vi "Update_Repeat_Param_Value_SubVI.vi"(10 "String":string, 11 "Experiment 6":T1) -> (3 "Experiment 5":T1)   [LabVIEW 2014]
uses:
  <userlib>/Nanonis Prog Interface V5/Scan/Grid/LinePatternGet.vi
  <userlib>/Nanonis Prog Interface V5/Scan/Grid/LinePatternSet.vi
  <userlib>/Nanonis Prog Interface V5/Nanonis Prog Interface.lvlib
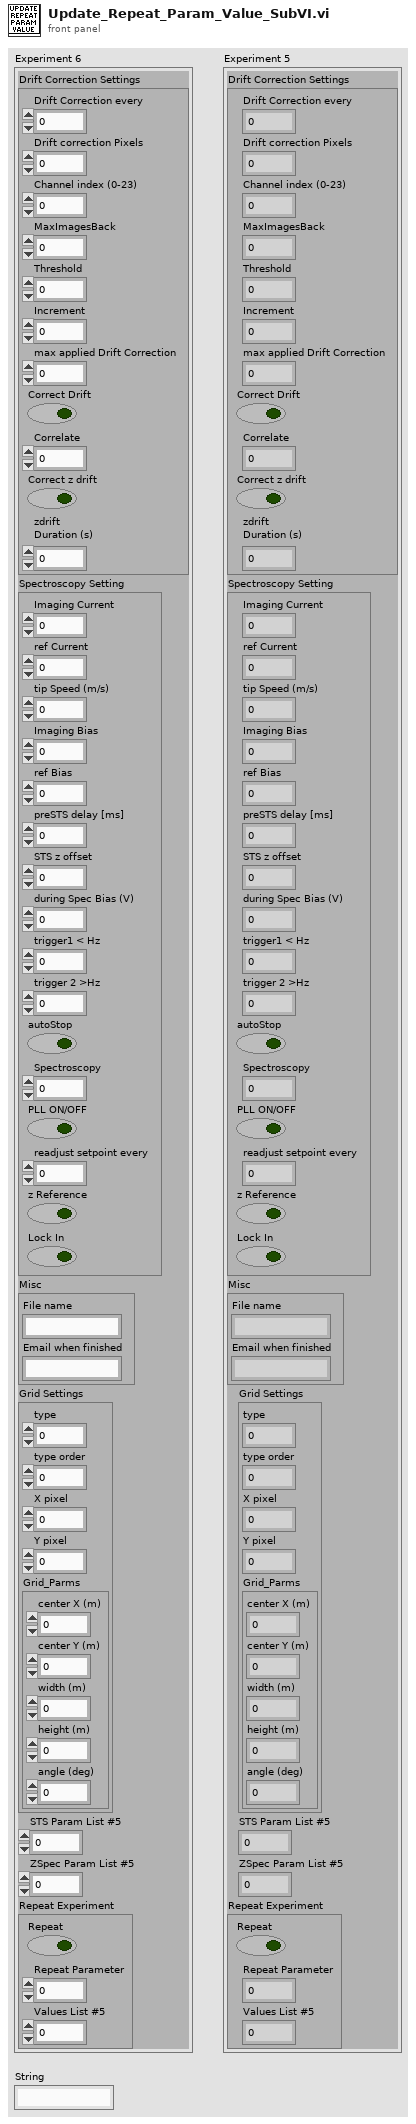
[diagram p1: front panel]
types:
  T1 = cluster{"Drift Correction Settings":cluster{"Drift Correction every":i32, "Drift correction Pixels":i32, "Channel index (0-23)":u8, "MaxImagesBack":i32, "Threshold":i32, "Increment":i32, "max applied Drift Correction":i32, "Correct Drift":bool, "Correlate":u16, "Correct z drift":bool, "zdrift \nDuration (s)":dbl}, "Spectroscopy Setting":cluster{"Imaging Current":dbl, "ref Current":dbl, "tip Speed (m/s)":sgl, "Imaging Bias":dbl, "ref Bias":dbl, "preSTS delay [ms]":u32, "STS z offset":dbl, "during Spec Bias (V)":sgl, "trigger1 < Hz":sgl, "trigger 2 >Hz":sgl, "autoStop":bool, "Spectroscopy":u16, "PLL ON/OFF":bool, "readjust setpoint every ":i32, "z Reference":bool, "Lock In":bool}, "Misc":cluster{"File name":string, "Email when finished":string}, "Grid Settings":cluster{"type":u16, "type order":u16, "X pixel":i32, "Y pixel":i32, "Grid_Parms":cluster{"center X (m)":sgl, "center Y (m)":sgl, "width (m)":sgl, "height (m)":sgl, "angle (deg)":sgl}}, "STS Param List #5 ":u16, "ZSpec Param List #5  ":u16, "Repeat Experiment":cluster{"Repeat":bool, "Repeat Parameter":u16, "Values List #5":i32}}
  T2 = cluster{"X (m)":sgl, "Y (m)":sgl, "Text":string, "Color":u32, "Visible":bool}[]
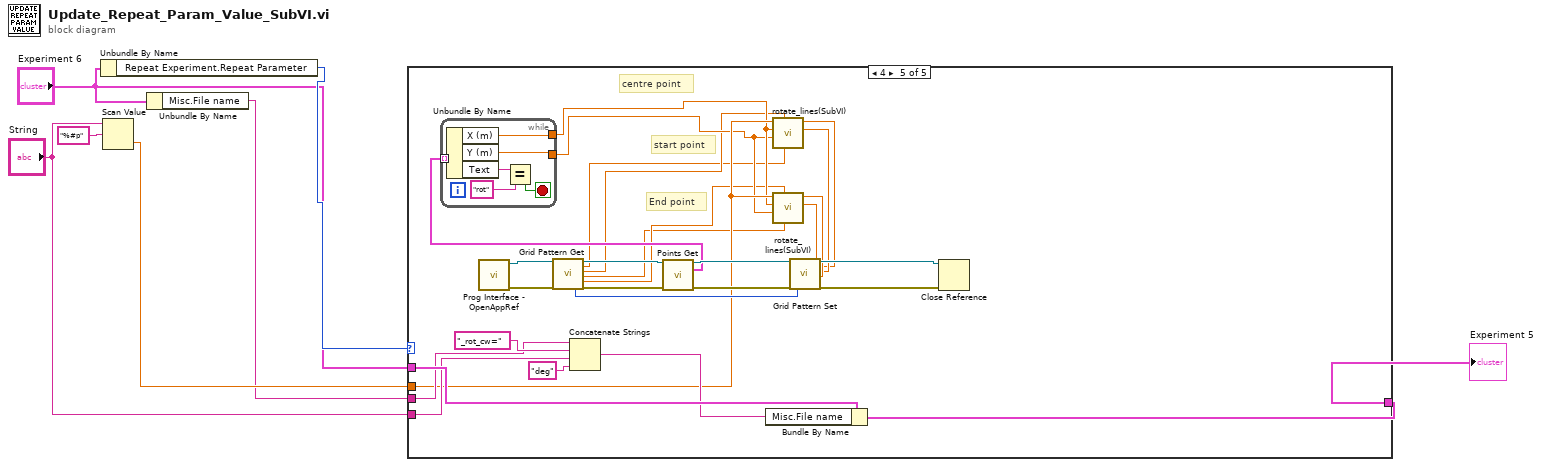
[diagram p0: block diagram]
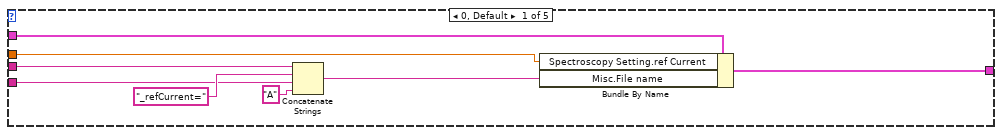
[diagram p2: hidden frame]
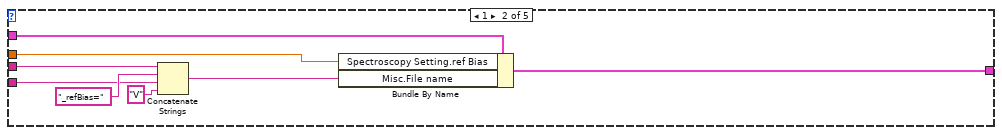
[diagram p3: hidden frame]
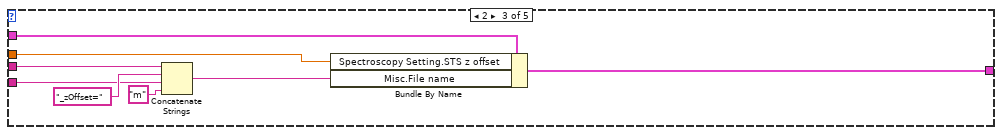
[diagram p4: hidden frame]
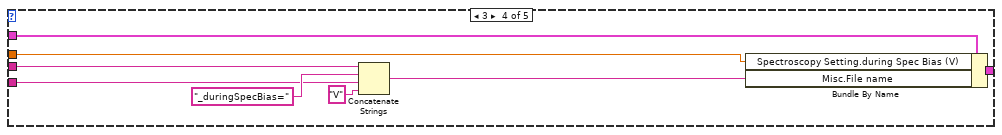
[diagram p5: hidden frame]
diagram:
  n1 = Unbundle By Name("Experiment 6") -> ("Repeat Experiment.Repeat Parameter"=w6:u16)
  n2 = Scan Value(string="String", format string="%#p") -> (value=w5:dbl)  [unwired: 1 in, 1 out]
  n3 = Unbundle By Name("Experiment 6") -> ("Misc.File name"=w2:string)
  n4 = case shown="4" w6 {
    tunnel: w5 -> [w15 w23 w31 w39 w46]
    tunnel: "Experiment 6" -> [w14 w22 w30 w38 w67]
    tunnel: [w13 w21 w29 w37 w66] -> w7
    tunnel: w2 -> [w12 w20 w28 w34 w63]
    tunnel: "String" -> [w10 w18 w25 w33 w62]
    frame 0, Default {
      n5 = Concatenate Strings(w12, "_refCurrent=", w10, "A") -> (w8:string)
      n6 = Bundle By Name(cluster=w14, "Spectroscopy Setting.ref Current"=w15, "Misc.File name"=w8) -> (w13:T1)
    }
    frame 1 {
      n7 = Concatenate Strings(w20, "_refBias=", w18, "V") -> (w16:string)
      n8 = Bundle By Name(cluster=w22, "Spectroscopy Setting.ref Bias"=w23, "Misc.File name"=w16) -> (w21:T1)
    }
    frame 2 {
      n9 = Concatenate Strings(w28, "_zOffset=", w25, "m") -> (w24:string)
      n10 = Bundle By Name(cluster=w30, "Spectroscopy Setting.STS z offset"=w31, "Misc.File name"=w24) -> (w29:T1)
    }
    frame 3 {
      n11 = Concatenate Strings(w34, "_duringSpecBias=", w33, "V") -> (w32:string)
      n12 = Bundle By Name(cluster=w38, "Spectroscopy Setting.during Spec Bias (V)"=w39, "Misc.File name"=w32) -> (w37:T1)
    }
    frame 4 {
      # "centre point"
      # "start point"
      # "End point"
      n13 = call <userlib>:"Prog Interface - OpenAppRef.vi"() -> ("Error out"=w58:errorcluster, "Application reference"=w59:refnum<vi>)  [unwired: 6 in]
      n14 = call-poly <userlib>:"Grid Pattern Get.vi"("Application ref in"=w59, "error in (no error)"=w58) -> ("Points"=w54:i32, "Application ref out"=w49:refnum<vi>, "Start X1 (m)"=w42:sgl, "Start Y1 (m)"=w43:sgl, "End X2 (m)"=w40:sgl, "End Y2 (m)"=w41:sgl, "error out"=w51:errorcluster)  [unwired: 11 in]
      n15 = Concatenate Strings(w63, "_rot_cw=", w62, "deg") -> (w61:string)
      n16 = call <userlib>:"Points Get.vi"("Application ref in"=w49, "error in (no error)"=w51) -> ("Application ref out"=w48:refnum<vi>, "Points"=w47:T2, "error out"=w50:errorcluster)  [unwired: 11 in]
      n17 = while {
        tunnel: [w73] -> _ mode=indexing
        tunnel: w47 -> [w73] mode=indexing
        tunnel: [w69] -> w45
        tunnel: [w68] -> w44
        stop <- w72 stop-if-true
        n18 = Unbundle By Name(w73) -> ("X (m)"=w69:sgl, "Y (m)"=w68:sgl, "Text"=w71:string)
        n19 = Equal?(x=w71, y="rot") -> (x = y?=w72:bool)
      }
      n20 = Bundle By Name(cluster=w67, "Misc.File name"=w61) -> (w66:T1)
      n21 = call "rotate_lines(SubVI).vi"("End X2 (m)"=w42, "End Y2 (m)"=w43, "centre Y1 (m)"=w44, "centre X1 (m)"=w45, "rotation in degrees"=w46) -> ("Rot End Y"=w53:dbl, "Rot End X"=w52:dbl)  [unwired: 5 in]
      n22 = call "rotate_lines(SubVI).vi"("End X2 (m)"=w40, "End Y2 (m)"=w41, "centre Y1 (m)"=w44, "centre X1 (m)"=w45, "rotation in degrees"=w46) -> ("Rot End Y"=w56:dbl, "Rot End X"=w55:dbl)  [unwired: 5 in]
      n23 = call-poly <userlib>:"Grid Pattern Set.vi"("Application ref in"=w48, "Start X1 (m)"=w52, "Start Y1 (m)"=w53, "End X2 (m)"=w55, "End Y2 (m)"=w56, "error in (no error)"=w50, "Points"=w54) -> ("Application ref out"=w60:refnum<vi>, "error out"=w57:errorcluster)  [unwired: 11 in]
      n24 = Close Reference(reference=w60, error in (no error)=w57) -> ()  [unwired: 1 out]
    }
  }
  "Experiment 5" <- w7
